vi "XML-String in Enum-Array.vi"(1 "XML-String":string) -> (0 "Enum-Objekte (N)":string[](array[string]))   [LabVIEW 2020, in "Anlagenuebersicht.lvlib" / "VisBx Anzeige.lvlib"]
uses:
  VisBx Anzeige.lvlib
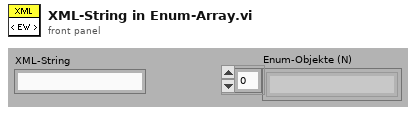
[diagram p1: front panel]
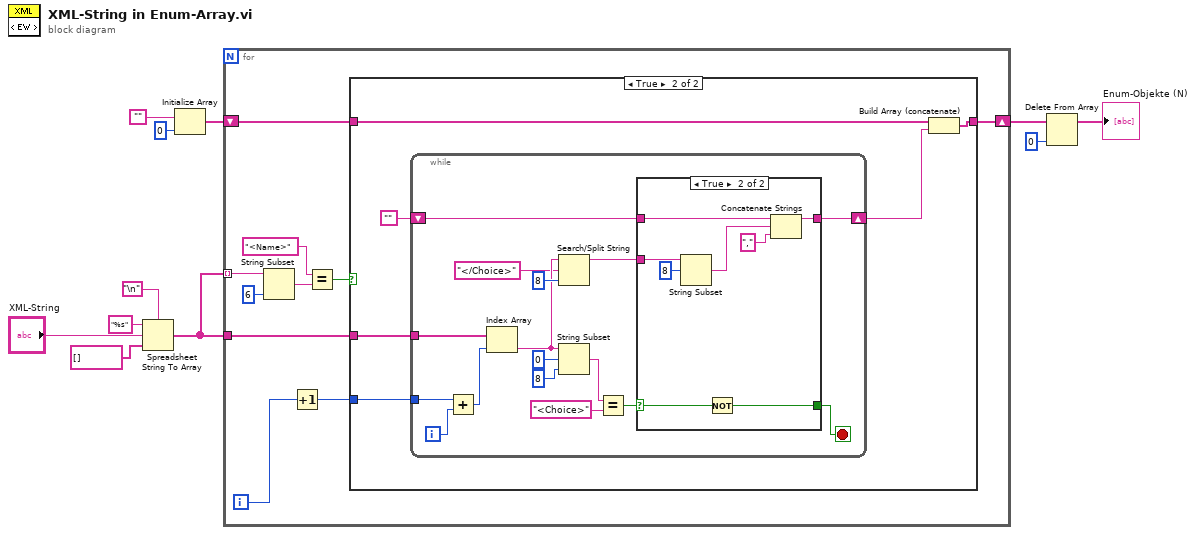
[diagram p0: block diagram]
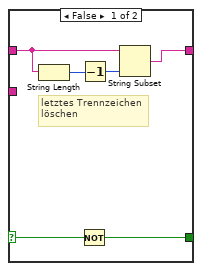
[diagram p3: hidden frame]
diagram:
  n1 = Spreadsheet String To Array(delimiter (Tab)="\n", format string="%s" ("Format-String"), spreadsheet string="XML-String", array type (2D Dbl)=string[] []) -> (array=w6:string[])
  n2 = Initialize Array("", 0 ("Dimension")) -> (w5:string[])
  n3 = for {
    tunnel: w6 -> [w21] mode=indexing
    tunnel: w6 -> [w18]
    shift-right: [w16] -> w3
    shift-left: w5 -> [w17]
    i -> [w15]
    n4 = String Subset(string=w21, length (rest)=6 ("Länge (Rest)")) -> (substring=w12:string)  [unwired: 1 out]
    n5 = Increment(x=w15) -> (x+1=w14:i32)
    n6 = Equal?(x="<Name>" ("y"), y=w12) -> (x = y?=w19:bool)
    n7 = case shown="True" w19 {
      tunnel: w18 -> [_ w26]
      tunnel: w17 -> [w22 w28]
      tunnel: [w22 w27] -> w16
      tunnel: w14 -> [_ w25]
      frame False {
      }
      frame True {
        n8 = while {
          tunnel: w26 -> [w37]
          tunnel: w25 -> [w39]
          shift-right: [w30] -> w23
          shift-left: "" -> [w31]
          i -> [w40]
          stop <- w29 stop-if-true
          n9 = Add(x=w39, y=w40) -> (x+y=w44:i32)
          n10 = Index Array(array=w37, index=w44) -> (element=w34:string)
          n11 = Search/Split String(string=w34, search string/char (-)="</Choice>" ("Nach String/Zeichen suchen (-)"), offset (0)=8 ("Offset (0)")) -> (substring before match=w32:string)  [unwired: 2 out]
          n12 = String Subset(string=w34, offset (0)=0 ("Offset (0)"), length (rest)=8 ("Länge (Rest)")) -> (substring=w42:string)
          n13 = Equal?(x=w42, y="<Choice>") -> (x = y?=w38:bool)
          n14 = case shown="True" w38 {
            selector: w38 -> [w50 w56]
            tunnel: w32 -> [_ w54]
            tunnel: w31 -> [w48 w58]
            tunnel: [w49 w57] -> w30
            tunnel: [w45 w55] -> w29
            frame False {
              # "letztes Trennzeichen\nlöschen"
              n15 = String Length(string=w48) -> (length=w47:i32)
              n16 = Not(x=w50) -> (.not. x?=w45:bool)
              n17 = Decrement(x=w47) -> (x-1=w46:i32)
              n18 = String Subset(string=w48, length (rest)=w46) -> (substring=w49:string)  [unwired: 1 out]
            }
            frame True {
              n19 = String Subset(string=w54, offset (0)=8 ("Offset (0)")) -> (substring=w53:string)  [unwired: 1 out]
              n20 = Not(x=w56) -> (.not. x?=w55:bool)
              n21 = Concatenate Strings(w58, w53, ",") -> (w57:string)
            }
          }
        }
        n22 = Build Array (concatenate)(w28, w23) -> (w27:string[])
      }
    }
  }
  n23 = Delete From Array(array=w3, index=0 ("Index")) -> (array with subset deleted=→"Enum-Objekte (N)":string[])  [unwired: 1 in, 1 out]
